vi "write file.vi"(8 "error in (no error)":errorcluster, 10 "Item Names":string[](array[string]), 11 "configuration file path":path) -> (0 "error out":errorcluster)   [LabVIEW 2020]
uses:
  <vilib>/Utility/config.llb/Write Key (String).vi
  <vilib>/Utility/config.llb/NI_LVConfig.lvlib
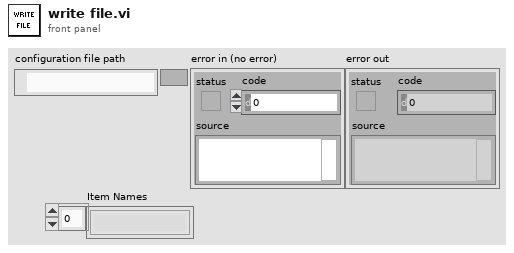
[diagram p1: front panel]
types:
  T1 = typedef "NI_LVConfig.lvlib/Config Data RefNum.ctl" = refnum<k1>
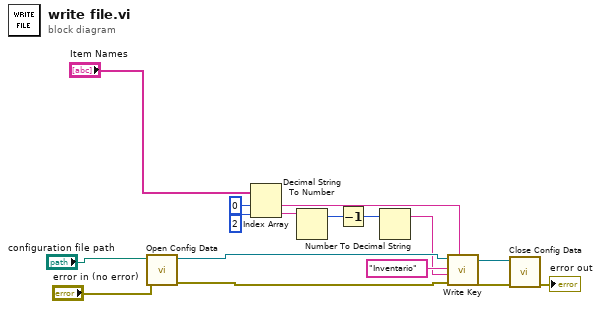
[diagram p0: block diagram]
diagram:
  n1 = call <vilib>:"Open Config Data.vi"("error in (no error)"="error in (no error)", "configuration file path"="configuration file path") -> ("error out"=w12:errorcluster, "refnum"=w13:T1)  [unwired: 7 in, 1 out]
  n2 = Index Array(array="Item Names", index #1=0 ("index"), index #2=2 ("index")) -> (element #1=w10:string, element #2=w6:string)
  n3 = Decimal String To Number(string=w6) -> (number=w5:i32)  [unwired: 2 in, 1 out]
  n4 = Decrement(x=w5) -> (x-1=w4:i32)
  n5 = Number To Decimal String(number=w4) -> (decimal integer string=w3:string)  [unwired: 1 in]
  n6 = call-poly <vilib>:"Write Key.vi"("section"=w10, "error in (no error)"=w12, "value"=w3, "key"="Inventario" ("section"), "refnum"=w13) -> ("error out"=w15:errorcluster, "refnum out"=w16:T1)  [unwired: 4 in, 1 out]
  n7 = call <vilib>:"Close Config Data.vi"("error in (no error)"=w15, "refnum"=w16) -> ("error out"=→"error out":errorcluster)  [unwired: 8 in, 1 out]
